vi "Teleop.vi"(10 "Match Info":T1={"Autonomous Elapsed Seconds"=0.0, "TeleOp Elapsed Seconds"=0.0, "Disabled Elapsed Seconds"=0.0, "Visited Autonomous"=FALSE, "Visited TeleOp"=FALSE, "Visited Disabled"=FALSE, "Autonomous Settings"={"Autonomous Style"=enum."Independent", "VI Refnum"=refnum}}, 11 "Call Context":T2) -> ()   [LabVIEW 2013]
doc: "This VI is called for each TeleOp packet received from the DS where the robot is not disabled. It is often used to read from the joysticks and update I/O or to update setpoints for timed control loops. It should complete and return within 20 milliseconds or it may miss DS packets."
uses:
  <vilib>/Rock Robotics/WPI/DriverStation/WPI_DriverStationDerivedRobotMode.ctl
  <vilib>/Rock Robotics/WPI/DriverStation/WPI_DriverStationMatch Info.ctl
  Robot Global Data.vi
  <vilib>/Rock Robotics/Network Tables/SD Read Number.vi
panel:
  in  "Optimum":dbl=10.0
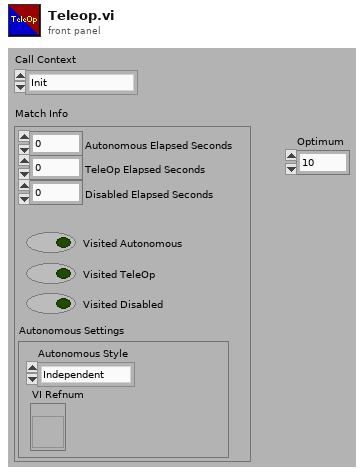
[diagram p1: front panel]
types:
  T1 = typedef "WPI_DriverStationMatch Info.ctl" = cluster{"Autonomous Elapsed Seconds":dbl, "TeleOp Elapsed Seconds":dbl, "Disabled Elapsed Seconds":dbl, "Visited Autonomous":bool, "Visited TeleOp":bool, "Visited Disabled":bool, "Autonomous Settings":cluster{"Autonomous Style":enum16{"Iterative", "Independent"}, "VI Refnum":refnum<vi>}}
  T2 = typedef "WPI_DriverStationDerivedRobotMode.ctl" = enum16{"Init", "Execute", "Stop"}
  T3 = typedef "WPI_JoystickButtonState.ctl" = cluster{"Button 1":bool, "Button 2":bool, "Button 3":bool, "Button 4":bool, "Button 5":bool, "Button 6":bool, "Button 7":bool, "Button 8":bool, "Button 9":bool, "Button 10":bool, "Button 11":bool, "Button 12":bool}
  T4 = cluster{"Axes":cluster{"X Axis":dbl, "Y Axis":dbl, "Throttle":dbl, "Unused":dbl, "Unused":dbl, "Unused":dbl}, "Buttons":T3}
  T5 = cluster{"Axes":cluster{"X Axis":dbl, "Y Axis":dbl, "Twist-Handle":dbl, "Throttle":dbl, "Unused":dbl, "Unused":dbl}, "Buttons":T3}
  T6 = cluster{"Axes":cluster{"Joystick 1":cluster{"X Axis":dbl, "Y Axis":dbl}, "Triggers":dbl, "Joystick 2":cluster{"X Axis":dbl, "Y Axis":dbl}}, "Buttons":T3}
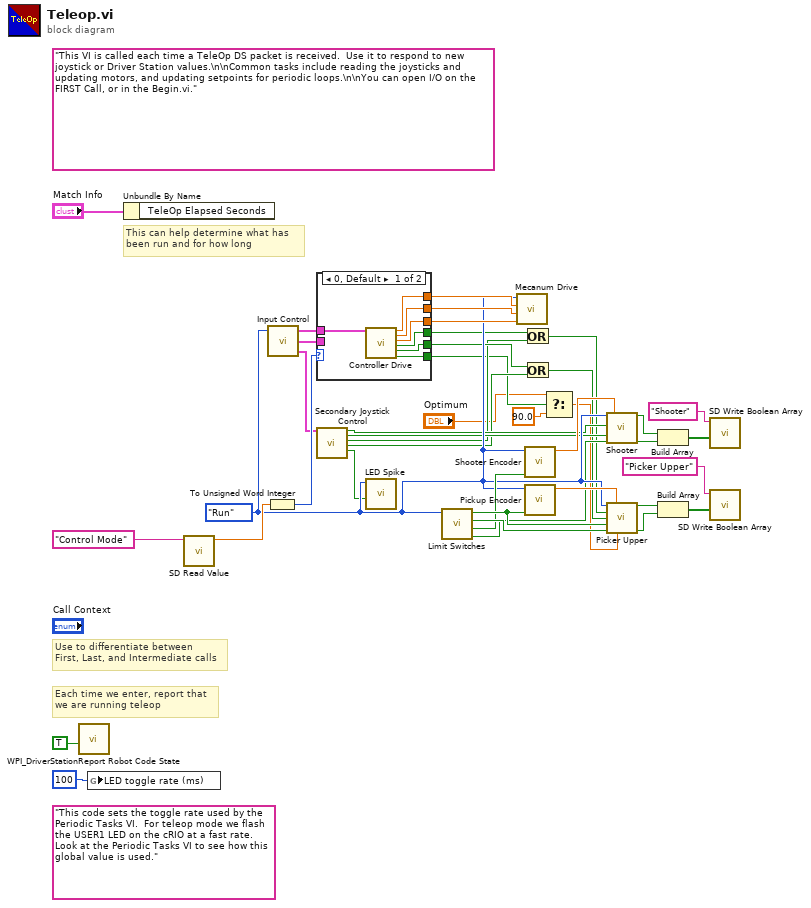
[diagram p0: block diagram]
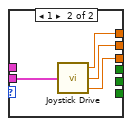
[diagram p2: hidden frame]
diagram:
  w24 = enum16{"Open", "Run", "End"}."Run" ("State")
  (unwired) "This code sets the toggle rate used by the Periodic Tasks VI.  For teleop mode we flash the USER1 LED on the cRIO at a fast rate.  Look at the Periodic Tasks VI to see how this global value is used."
  (unwired) "This VI is called each time a TeleOp DS packet is received.  Use it to respond to new joystick or Driver Station values.\n\nCommon tasks include reading the joysticks and updating motors, and updating setpoints for periodic loops.\n\nYou can open I/O on the FIRST Call, or in the Begin.vi."
  # "Each time we enter, report that\nwe are running teleop"
  # "Use to differentiate between\nFirst, Last, and Intermediate calls"
  # "This can help determine what has\nbeen run and for how long"
  n1 = call <vilib>:"WPI_DriverStationReport Robot Code State.vi"("TeleOp"=TRUE ("Autonomous")) -> ()  [unwired: 10 in, 1 out]
  n2 = global write "Robot Global Data.vi" "LED toggle rate (ms)"(u32 100 ("LED ms toggle rate")) -> ()
  n3 = Unbundle By Name("Match Info") -> ()  [unwired: 1 out]
  n4 = call-poly <vilib>:"SD Read Value.vi"("Name"="Control Mode") -> ("Numeric"=w36:dbl)  [unwired: 8 in, 2 out]
  n5 = To Unsigned Word Integer(number=w36) -> (unsigned 16bit integer=w35:u16)
  n6 = call "Input Control.vi"("State"=w24) -> ("Secondary Joystick"=w22:T4, "Twist-handle Joystick"=w27:T5, "Gamepad"=w34:T6)  [unwired: 2 in]
  n7 = case shown="0, Default" w35 {
    tunnel: w34 -> [w47 _]
    tunnel: [w46 w50] -> w33
    tunnel: [w45 w49] -> w32
    tunnel: [w44 w48] -> w31
    tunnel: [w43 _] -> w14
    tunnel: [w42 _] -> w17
    tunnel: w27 -> [_ w51]
    tunnel: [w41 _] -> w4
    frame 0, Default {
      n8 = call "Controller Drive.vi"("input cluster"=w47) -> ("Strafe"=w46:dbl, "Forward/Reverse"=w45:dbl, "Turn"=w44:dbl, "Picker Upper Up"=w43:bool, "Picker Upper Down"=w42:bool, "Breakpoint"=w41:bool)  [unwired: 13 in]
    }
    frame 1 {
      n9 = call "Joystick Drive.vi"("Joystick Drive"=w51) -> ("Strafe"=w50:dbl, "Forward/Backward"=w49:dbl, "Turn"=w48:dbl)
    }
  }
  n10 = call "Secondary Joystick Control.vi"("Secondary Joystick"=w22) -> ("Shooter return"=w21:bool, "Shooter 4 feet"=w20:bool, "Picker upper up"=w15:bool, "Picker upper down"=w18:bool, "LED"=w19:bool)  [unwired: 14 in]
  n11 = call "LED Spike.vi"("ON/OFF"=w19, "State"=w24) -> ()  [unwired: 10 in]
  n12 = call "Limit Switches.vi"("State Control"=w24) -> ("Shooter Top"=w23:bool, "Shooter Bottom"=w26:bool, "Picker Upper Bottom"=w28:bool, "Picker Upper Top"=w29:bool)  [unwired: 7 in]
  n13 = call "Mecanum Drive.vi"("Turn"=w31, "Forward/Backward"=w32, "Strafe"=w33, "State Control"=w24) -> ()  [unwired: 4 in]
  n14 = Or(x=w14, y=w15) -> (x .or. y?=w13:bool)
  n15 = Or(x=w17, y=w18) -> (x .or. y?=w16:bool)
  n16 = call "Shooter Encoder.vi"("Reset Encoder?"=w26, "State Control"=w24) -> ("Encoder Degrees"=w25:dbl)  [unwired: 2 in, 3 out]
  n17 = call "Pickup Encoder.vi"("Reset Encoder?"=w29, "State Control"=w24) -> ("Encoder Degrees"=w30:dbl)  [unwired: 2 in, 3 out]
  n18 = Select(t="Optimum", s=w4, f=90.0) -> (s? t:f=w1:dbl)
  n19 = call "Shooter.vi"("State Control"=w24, "Return"=w21, "4 ft"=w20, "Top Limit"=w23, "Encoder"=w25) -> ("Fully shot?"=w12:bool, "Fully retracted?"=w11:bool)  [unwired: 13 in]
  n20 = call "Picker Upper.vi"("State Control"=w24, "Encoder"=w30, "Up"=w13, "Down"=w16, "Top limit"=w29, "Bottom Limit"=w28, "Down break"=w1) -> ("Fully up?"=w8:bool, "Fully down?"=w7:bool)  [unwired: 7 in]
  n21 = Build Array(w12, w11) -> (w10:bool[])
  n22 = Build Array(w8, w7) -> (w6:bool[])
  n23 = call <vilib>:"SD Write Boolean Array.vi"("Boolean Array"=w10, "Name"="Shooter") -> ()  [unwired: 8 in, 2 out]
  n24 = call <vilib>:"SD Write Boolean Array.vi"("Boolean Array"=w6, "Name"="Picker Upper") -> ()  [unwired: 8 in, 2 out]
